vi "Example - Authenticate using WAMP-SCRAM.vi"() -> ()   [LabVIEW 2020, in "wamplv.lvlib"]
uses:
  wamplv.lvlib
  WAMP Client/WAMP Client.lvclass/WAMP Client.ctl
  WAMP Client/API/WAMP/Publish.vi/5e405bcd-0c6d-46be-a87b-06ec174a83c2.vi
  WAMP Client/API/WAMP/Publish (async).vi
  WAMP Client/Private/SubVIs/Raise Internal Message.vi
  WAMP Client/API/WAMP/Publish (async).vi/56cb05c7-ccfa-42e5-a428-2bd237dbc257.vi
  WAMP Client/Private/Authentication/Add WAMP-SCRAM authenticator.vi
  <vilib>/Utility/error.llb/Error Cluster From Error Code.vi
  WAMP Client/WAMP Client.lvclass
panel:
  in  "Unhashed Client Key":string="testclientkey"
  in  "Ticket (e.g. password)":string="secret"
  in  "Authorisation ID (e.g.username)":string="foobar@example.com"
  in  "Arguments":string
  in  "Topic URI":string="test.topic"
  in  "Realm":string="realm1"
  in  "Router URL":string="ws://192.168.1.10:8080/ws"
  # "Example: authenticate sign-in WAMP-SCRAM and publish"
  # "Note: wamplv only supports PBKDF2 with WAMP-SCRAM. \nWAMP-SCRAM is experimental and may not work with \nyour router."
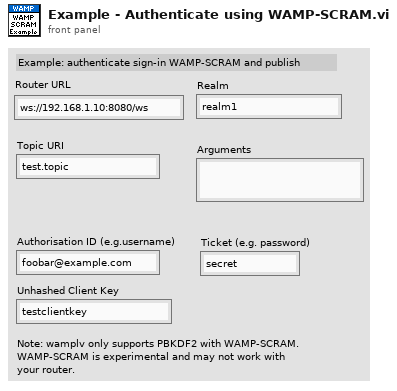
[diagram p1: front panel]
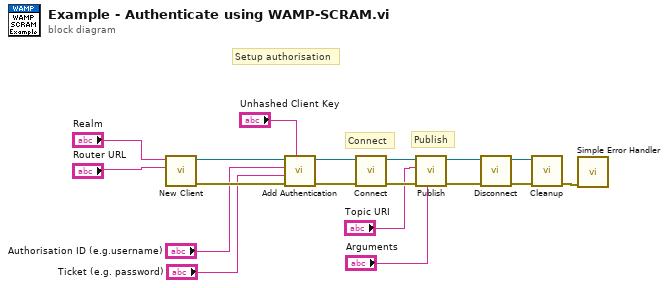
[diagram p0: block diagram]
diagram:
  # "Setup authorisation"
  # "Publish"
  # "Connect"
  n1 = call "New Client.vi"("Address"="Router URL", "Realm"="Realm") -> ("error out"=w6:errorcluster, "WAMP client out"=w7:refnum<class "WAMP Client.lvclass">)  [unwired: 8 in]
  n2 = call-poly "Add Authentication.vi"("Client Key"="Unhashed Client Key", "error in (no error)"=w6, "Secret"="Ticket (e.g. password)", "Authentication ID"="Authorisation ID (e.g.username)", "WAMP Client in"=w7) -> ("error out"=w4:errorcluster, "WAMP Client out"=w5:refnum<class "WAMP Client.lvclass">)  [unwired: 5 in]
  n3 = call "Connect.vi"("error in"=w4, "WAMP Client in"=w5) -> ("error out"=w11:errorcluster, "WAMP Client out"=w13:refnum<class "WAMP Client.lvclass">)  [unwired: 8 in]
  n4 = call "Publish.vi"("Arguments"="Arguments", "Error in"=w11, "Topic"="Topic URI", "WAMP Client in"=w13) -> ("Error out"=w10:errorcluster, "WAMP Client out"=w12:refnum<class "WAMP Client.lvclass">)  [unwired: 5 in, 1 out]
  n5 = call-dynamic "Disconnect.vi"("error in"=w10, "WAMP Client in"=w12) -> ("error out"=w14:errorcluster, "WAMP Client out"=w16:refnum<class "WAMP Client.lvclass">)  [unwired: 8 in]
  n6 = call-dynamic "Cleanup.vi"("error in"=w14, "WAMP Client in"=w16) -> ("error out"=w15:errorcluster)  [unwired: 8 in, 1 out]
  n7 = call <vilib>:"Simple Error Handler.vi"("error in (no error)"=w15) -> ()  [unwired: 4 in, 5 out]
